vi "module-09-analog-rate-calc.vi"() -> ()   [LabVIEW 2019]
uses:
  samples-common-library/Ctrl_Training_Library_Protected/CtrlTrain_Analog_HighSelect.vi
  <vilib>/Rock Robotics/WPI/ThirdParty/JAS_Junk/TrajLib/LinearFilter_ResetToValue.vi
  <vilib>/Rock Robotics/WPI/ThirdParty/JAS_Junk/TrajLib/LinearFilter_Calculate.vi
  <vilib>/Rock Robotics/WPI/ThirdParty/JAS_Junk/TrajLib/Util_GetTime.vi
  <vilib>/Rock Robotics/WPI/ThirdParty/JAS_Junk/TrajLib/LinearFilter_MovingAverage.vi
  <vilib>/Rock Robotics/WPI/ThirdParty/JAS_Junk/TrajLib/LinearFilter_LowPassBW1.vi
  <vilib>/Rock Robotics/WPI/ThirdParty/JAS_Junk/TrajLib/LinearFilter_LowPassBW2.vi
  <vilib>/Rock Robotics/WPI/ThirdParty/JAS_Junk/TrajLib/LinearFilter_HighPassBW1.vi
  <vilib>/Rock Robotics/WPI/ThirdParty/JAS_Junk/TrajLib/LinearFilter_HighPassBW2.vi
  samples-common-library/Ctrl_Training_Library_Protected/CtrlTrainingLibary_Protected.lvlib
  <vilib>/Rock Robotics/WPI/ThirdParty/JAS_Junk/TrajLib/Trajectory_Library.lvlib
panel:
  in  "Tab Control":enum32{"Control Panel", "Logic"}(tab)
  in  "Noise Gain":dbl=1.0
  in  "Auto Generate\nInput":bool
  out "Input Auto\nGenerated":bool
  out "Rate of Rate \n(units/Sec/Sec)\nex: Acceleration":dbl
  out "Rate (units/Sec)\nex: Speed":dbl
  in  "Input\n (ex:\n Distance)":dbl(slide)=10.0 scale=-100.0..100.0
  in  "Enable Noise":bool
  out "Trend":T1(graph)
  out "Noise Enabled":bool
  out "Filtered Rate (units/Sec)\nex: Speed":dbl
  out "Filtered Rate of Rate \n(units/Sec/Sec)\nex: Acceleration 2":dbl
  # "Rate Calc Test"
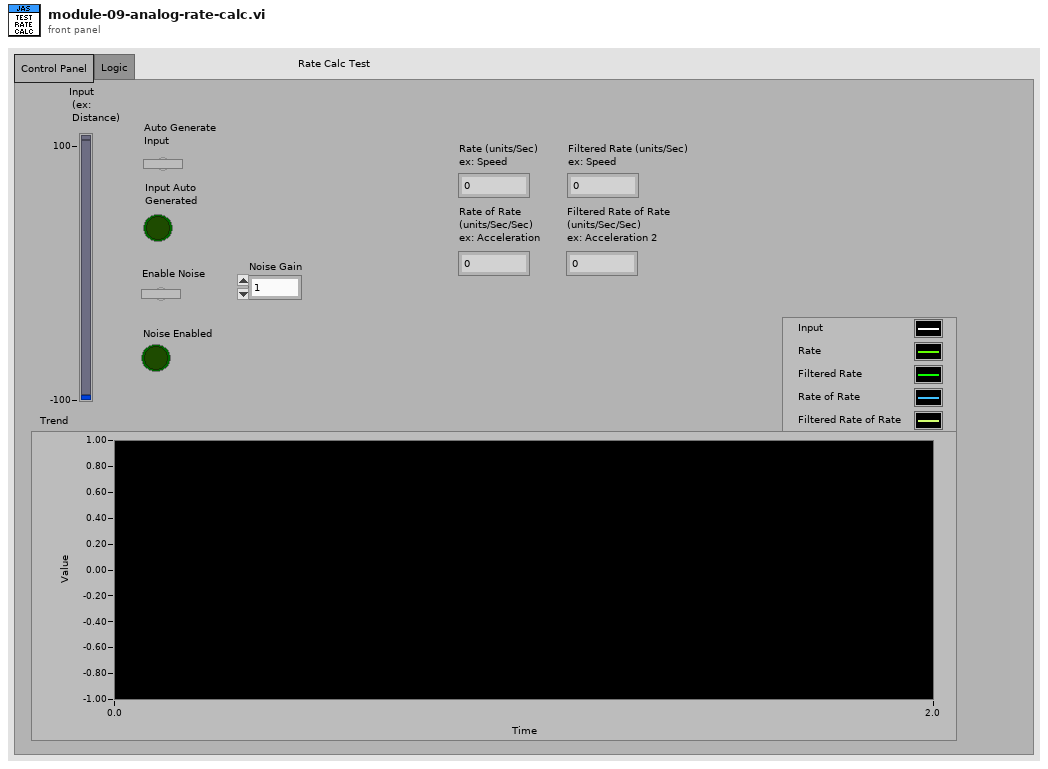
[diagram p1: front panel]
types:
  T1 = cluster{dbl, "Output":dbl, "Value_Output":dbl, "Output":dbl, "Value_Output":dbl}
  T2 = enum16{"Moving Average", "Low Pass 1st Order Butterworth", "Low Pass 2nd Order Butterworth", "High Pass 1st Order Butterworth", "High Pass 2nd Order Butterworth"}
  T3 = cluster{dbl, "Output":dbl, "Output":dbl, "Output":dbl, "Output":dbl}
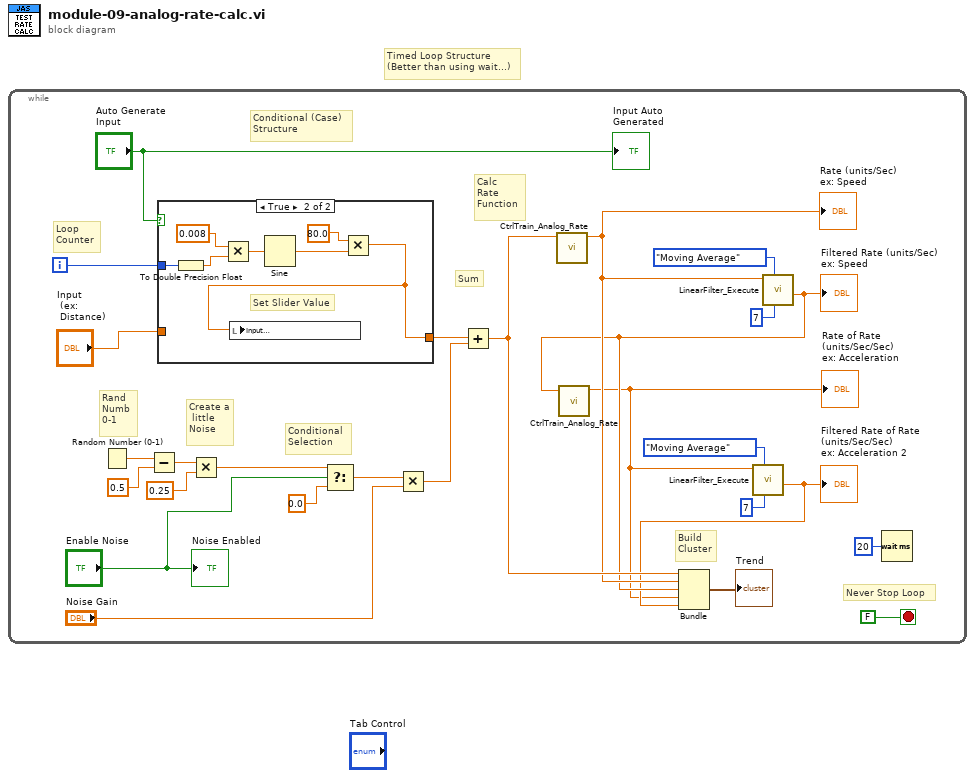
[diagram p0: block diagram]
diagram:
  # "Timed Loop Structure\n(Better than using wait...)"
  n1 = while {
    i -> [w14]
    stop <- FALSE stop-if-true
    # "Conditional (Case)\nStructure"
    # "Create a\n little\nNoise"
    # "Rand\nNumb\n0-1"
    # "Conditional\nSelection"
    # "Calc\nRate\nFunction"
    # "Sum"
    # "Build\nCluster"
    # "Loop \nCounter"
    # "Never Stop Loop"
    n2 = Random Number (0-1)() -> (number: 0 to 1=w24:dbl)
    n3 = Subtract(x=w24, y=0.5) -> (x-y=w22:dbl)
    n4 = case shown="True" "Auto Generate\nInput" {
      tunnel: "Input\n (ex:\n Distance)" -> [w27 _]
      tunnel: [w27 w28] -> w15
      tunnel: w14 -> [_ w34]
      frame False {
      }
      frame True {
        # "Set Slider Value"
        n5 = To Double Precision Float(number=w34) -> (double precision float=w33:dbl)
        n6 = Multiply(x=0.008, y=w33) -> (x*y=w31:dbl)
        n7 = Sine(x=w31) -> (sin(x)=w30:dbl)
        n8 = Multiply(x=80.0 ("y"), y=w30) -> (x*y=w28:dbl)
        n9 = local write "Input\n (ex:\n Distance)"(w28) -> ()
      }
    }
    n10 = Multiply(x=w22, y=0.25) -> (x*y=w20:dbl)
    n11 = Select(t=w20, s="Enable Noise", f=0.0) -> (s? t:f=w3:dbl)
    n12 = Multiply(x=w3, y="Noise Gain") -> (x*y=w1:dbl)
    n13 = Add(x=w15, y=w1) -> (x+y=w18:dbl)
    n14 = call "CtrlTrain_Analog_Rate.vi"("Input"=w18) -> ("Output"=w9:dbl)  [unwired: 10 in]
    "Rate (units/Sec)\nex: Speed" <- w9
    n15 = call <vilib>:"LinearFilter_Execute.vi"("Samples"=7, "Filter Type"=T2."Moving Average", "Input"=w9) -> ("Output"=w8:dbl)  [unwired: 7 in, 1 out]
    "Filtered Rate (units/Sec)\nex: Speed" <- w8
    n16 = call "CtrlTrain_Analog_Rate.vi"("Input"=w8) -> ("Output"=w4:dbl)  [unwired: 10 in]
    "Rate of Rate \n(units/Sec/Sec)\nex: Acceleration" <- w4
    n17 = call <vilib>:"LinearFilter_Execute.vi"("Samples"=7, "Filter Type"=T2."Moving Average", "Input"=w4) -> ("Output"=w5:dbl)  [unwired: 7 in, 1 out]
    "Filtered Rate of Rate \n(units/Sec/Sec)\nex: Acceleration 2" <- w5
    n18 = Bundle(w18, "Output"=w9, "Output"=w8, "Output"=w4, "Output"=w5) -> (→"Trend":T3)  [unwired: 1 in]
    n19 = Wait (ms)(milliseconds to wait=u32 20) -> ()  [unwired: 1 out]
    "Noise Enabled" <- "Enable Noise"
    "Input Auto\nGenerated" <- "Auto Generate\nInput"
  }
